vi "Untitled 1.vi"() -> ()   [LabVIEW 2018]
panel:
  in  "Blank Button":bool
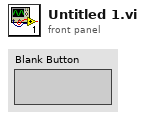
[diagram p1: front panel]
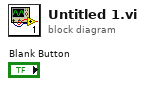
[diagram p0: block diagram]
diagram:
